vi "8-bit video export-AVI read by mode.vi"(7 "Frame number (unity-based)":i32=1 min=1, 8 "error in (no error)":errorcluster, 9 "RGB image ref in":T4, 11 "AVI modes refs":T1) -> (0 "error out":errorcluster, 1 "RGB image ref out":T4, 3 "AVI modes refs":T1)   [LabVIEW 2013]
uses:
  <vilib>/vision/Image Controls.llb/IMAQ Image.ctl
  Typedefs/AVI modes refs cluster.ctl
  <vilib>/vision/Avi1.llb/AviRefnum.ctl
  <vilib>/vision/Avi.llb/IMAQ AVI2 Refnum.ctl
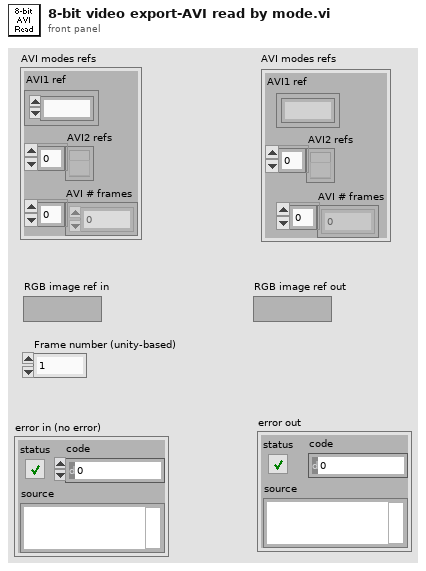
[diagram p1: front panel]
types:
  T1 = typedef "AVI modes refs cluster.ctl" = cluster{"AVI1 ref":T2, "AVI2 refs":T3[], "AVI # frames":u32[]}
  T2 = typedef "AviRefnum.ctl" = refnum<k1>
  T3 = typedef "IMAQ AVI2 Refnum.ctl" = refnum<k20>
  T4 = typedef "IMAQ Image.ctl" = refnum<image>
  T5 = typedef "AVI implementation enum.ctl" = enum16{"AVI1", "AVI2"}
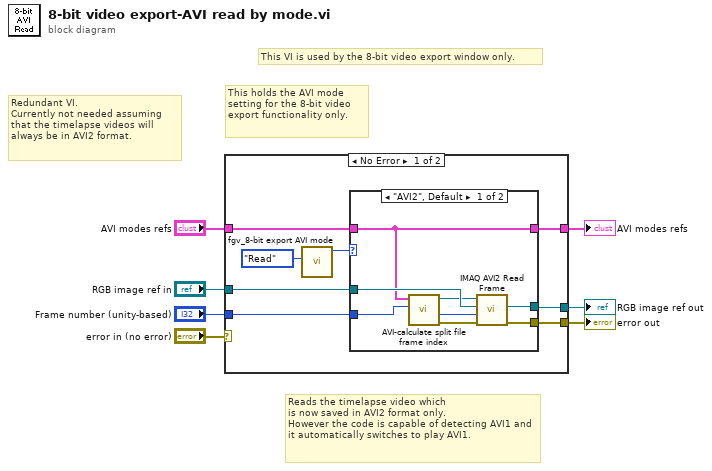
[diagram p0: block diagram]
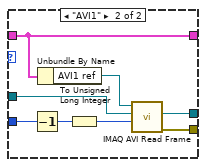
[diagram p2: hidden frame]
diagram:
  # "Redundant VI.\nCurrently not needed assuming that the timelapse videos will always be in AVI2 format."
  # "This VI is used by the 8-bit video export window only."
  # "This holds the AVI mode setting for the 8-bit video export functionality only."
  # "Reads the timelapse video which \nis now saved in AVI2 format only.\nHowever the code is capable of detecting AVI1 and it automatically switches to play AVI1."
  n1 = case shown="No Error" "error in (no error)" {
    selector: "error in (no error)" -> [_ w34]
    tunnel: [w15 w33] -> w7
    tunnel: "RGB image ref in" -> [w14 w33]
    tunnel: "AVI modes refs" -> [w13 w32]
    tunnel: [w12 w32] -> w4
    tunnel: [w11 w34] -> w3
    tunnel: "Frame number (unity-based)" -> [w10 _]
    frame No Error {
      n2 = call "fgv_8-bit export AVI mode.vi"("Function"=enum16{"Intialize", "Write", "Read", "Clear"}."Read") -> ("AVI mode"=w8:T5)  [unwired: 9 in, 1 out]
      n3 = case shown="\"AVI2\", Default" w8 {
        tunnel: [w21 w31] -> w11
        tunnel: [w23 w30] -> w15
        tunnel: w13 -> [w16 w24]
        tunnel: w14 -> [w22 w29]
        tunnel: [w16 w24] -> w12
        tunnel: w10 -> [w17 w26]
        frame "AVI2", Default {
          n4 = call "AVI-calculate split file frame index.vi"("Frame number (unity-based) in"=w17, "AVI modes refs"=w16) -> ("error out"=w19:errorcluster, "Index of frame in split file"=w20:u32, "AVI2 split file ref"=w18:T3)  [unwired: 6 in, 1 out]
          n5 = call "IMAQ AVI2 Read Frame"("error in (no error)"=w19, "Frame Number"=w20, "Image"=w22, "AVI Refnum"=w18) -> ("error out"=w21:errorcluster, "Image Out"=w23:T4)  [unwired: 5 in, 1 out]
        }
        frame "AVI1" {
          n6 = Decrement(x=w26) -> (x-1=w25:i32)
          n7 = Unbundle By Name(w24) -> ("AVI1 ref"=w28:T2)
          n8 = To Unsigned Long Integer(number=w25) -> (unsigned 32bit integer=w27:u32)
          n9 = call "IMAQ AVI Read Frame"("Frame Number"=w27, "Image"=w29, "Avi Refnum"=w28) -> ("error out"=w31:errorcluster, "Image Out"=w30:T4)  [unwired: 5 in, 2 out]
        }
      }
    }
    frame Error {
    }
  }
  "RGB image ref out" <- w7
  "error out" <- w3
  "AVI modes refs" <- w4
